vi "Add Offset and Mask to Image.vi"(5 "y":i32, 6 "x":i32, 7 "Image In":T1) -> (3 "Image Out":T1)   [LabVIEW 2025, in "XNode Support.lvlib"]
uses:
  XNode Support.lvlib
  <vilib>/picture/picture.llb/imagedata.ctl
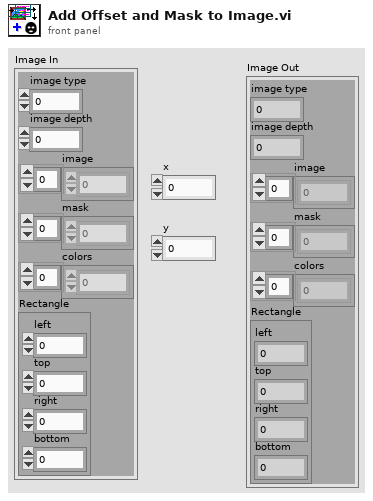
[diagram p1: front panel]
types:
  T1 = typedef "imagedata.ctl" = cluster{"image type":i32, "image depth":i32, "image":u8[], "mask":u8[], "colors":u32[], "Rectangle":cluster{"left":i16, "top":i16, "right":i16, "bottom":i16}}
  T2 = cluster{"left":i16, "top":i16, "right":i16, "bottom":i16}
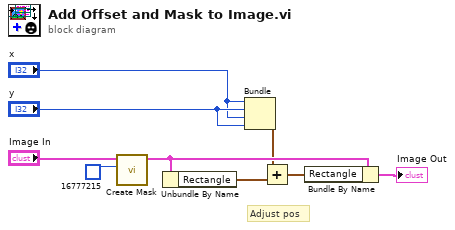
[diagram p0: block diagram]
diagram:
  # "Adjust pos"
  n1 = call <vilib>:"Create Mask.vi"("Mask Color (Black)"=u32 16777215, "image data"="Image In") -> ("image data"=w9:T1)  [unwired: 9 in]
  n2 = Unbundle By Name(w9) -> ("Rectangle"=w5:T2)
  n3 = Bundle("x"="x", "y"="y", "x"="x", "y"="y") -> (w4:cluster{"x":i32, "y":i32, "x":i32, "y":i32})  [unwired: 1 in]
  n4 = Add(x=w4, y=w5) -> (x+y=w6:cluster{i32, i32, i32, i32})
  n5 = Bundle By Name(cluster=w9, "Rectangle"=w6) -> (→"Image Out":T1)
